vi "AddSequenceRunReference.vi"(8 "error in":errorcluster, 10 "Id":string, 11 "OperationRun in":refnum<class "OperationRun.lvclass">) -> (0 "error out":errorcluster, 2 "SequenceRun":refnum<class "SequenceRunReference.lvclass">, 3 "OperationRun out":refnum<class "OperationRun.lvclass">)   [LabVIEW 2021, in "ProligentXMLGenerator.lvlib" / "OperationRun.lvclass"]
doc: "Add an OperationRun.\n\nDefines the operation run, a logical container for the execution of sequences and processes.\nOperation runs are globaly unique by their OperationRunId property."
uses:
  OperationRun.lvclass
  OperationRun.lvclass/OperationRun.ctl
  SequenceRun/SequenceRunReference/SequenceRunReference.lvclass
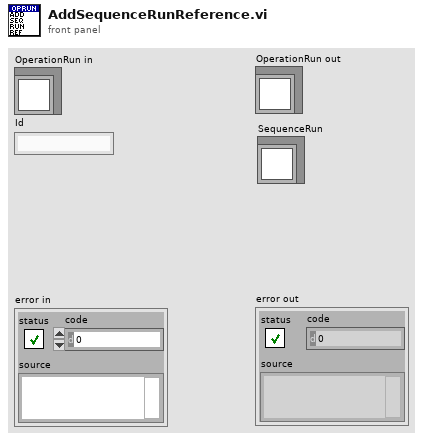
[diagram p1: front panel]
types:
  T1 = typedef "ProligentXMLGenerator.lvlib/OperationRun.lvclass/Data.ctl" = cluster{"Name":string, "Characteristics":refnum<class "Characteristic.lvclass">[], "Documents":refnum<class "Document.lvclass">[], "SequenceRuns":refnum<class "SequenceRun.lvclass">[], "FailureReferences":refnum<class "FailureReference.lvclass">[], "SequenceRunReferences":refnum<class "SequenceRunReference.lvclass">[], "CustomData":refnum<class "CustomData.lvclass">, "OperationRunId":refnum<class "Guid.lvclass">, "ProcessFullName":refnum<class "ProcessFullName.lvclass">, "ProcessVersion":refnum<class "NonEmptyString_64.lvclass">, "OperationName":refnum<class "NonEmptyString_65.lvclass">, "StationFullName":refnum<class "FullName.lvclass">, "User":refnum<class "NonEmptyString_255.lvclass">, "CallingOperationRunId":refnum<class "Guid.lvclass">, "OperationStatus":refnum<class "ExecutionStatus.lvclass">, "OperationRunStartTime":refnum<class "DateTime.lvclass">, "OperationRunEndTime":refnum<class "DateTime.lvclass">, "TimeZoneInfoId":string}
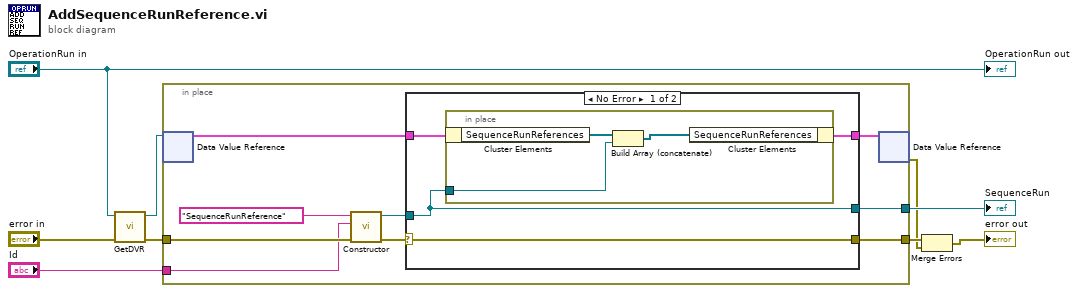
[diagram p0: block diagram]
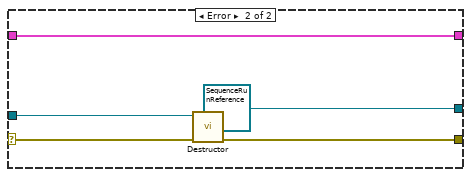
[diagram p2: hidden frame]
diagram:
  n1 = call "GetDVR.vi"("error in"="error in", "OperationRun"="OperationRun in") -> ("error out"=w3:errorcluster, "DVRReference"=w2:refnum<data-value>)  [unwired: 8 in]
  n2 = in-place "In Place Element Structure" {
    in-place-border: "Id" -> [w10]
    in-place-border: [w17] -> w4
    in-place-border: w3 -> [w16]
    in-place-border: [w13] -> w5
    n3 = in-place-dvr #1(w2) -> (w15:T1)  [unwired: 1 out]
    n4 = call "Constructor.vi"("error in"=w16, "Id"=w10, "Name"="SequenceRunReference") -> ("error out"=w18:errorcluster, "SequenceRunReference out"=w12:refnum<class "SequenceRunReference.lvclass">)  [unwired: 7 in]
    n5 = case shown="No Error" w18 {
      selector: w18 -> [w22 w29]
      tunnel: [w19 w30] -> w14
      tunnel: [w22 w28] -> w17
      tunnel: w12 -> [w21 w27]
      tunnel: w15 -> [w20 w30]
      tunnel: [w21 refnum<class "SequenceRunReference.lvclass"> refnum ("ProligentResultProcessor:SequenceRunReference")] -> w13
      frame No Error {
        n6 = in-place "In Place Element Structure" {
          in-place-border: w21 -> [w25]
          n7 = in-place-cluster #2(w20) -> ("SequenceRunReferences"=w24:refnum<class "SequenceRunReference.lvclass">[])
          n8 = Build Array (concatenate)(w24, w25) -> (w23:refnum<class "SequenceRunReference.lvclass">[])
          n9 = in-place-cluster #2("SequenceRunReferences"=w23) -> (w19:T1)
        }
      }
      frame Error {
        n10 = call "Destructor.vi"("error in"=w29, "SequenceRunReference in"=w27) -> ("error out"=w28:errorcluster)  [unwired: 9 in]
      }
    }
    n11 = in-place-dvr #1(w14) -> (w1:errorcluster)  [unwired: 1 out]
  }
  "SequenceRun" <- w5
  n12 = Merge Errors(w4, w1) -> (→"error out":errorcluster)
  "OperationRun out" <- "OperationRun in"
